vi "loadHTOutcount1.vi"(11 "file (use dialog)":path=path "C:/temp/ht/MachineState/MachineState.txt") -> ()   [LabVIEW 2012]
uses:
  <vilib>/addons/database/Connection.llb/DB Tools Open Connec (Path).vi
  <vilib>/Utility/file.llb/Read From Spreadsheet File (string).vi
  <vilib>/addons/database/Connection.llb/Conn Execute.vi
  <vilib>/addons/database/Recordset.llb/Rec Fetch Integer Data (R).vi
  <vilib>/addons/database/Recordset.llb/Rec Destroy - Connection.vi
  <vilib>/addons/database/NI_Database_API.lvlib
panel:
  out "ToRunSite":string
  out "concatenated string":string
  out "error out 2":errorcluster
  out "SQLDateTime 2":string
  in  "input cluster":T1
  out "output cluster":T1
  out "SQLDateTime":string
  out "time stamp":timestamp
  out "all rows":string[][](array[string])
  out "size(s)":i32[](array[numeric])
  out "error out":errorcluster
  out "output cluster 2":T2
  in  "input cluster 2":T2
  out "before substring 5":string
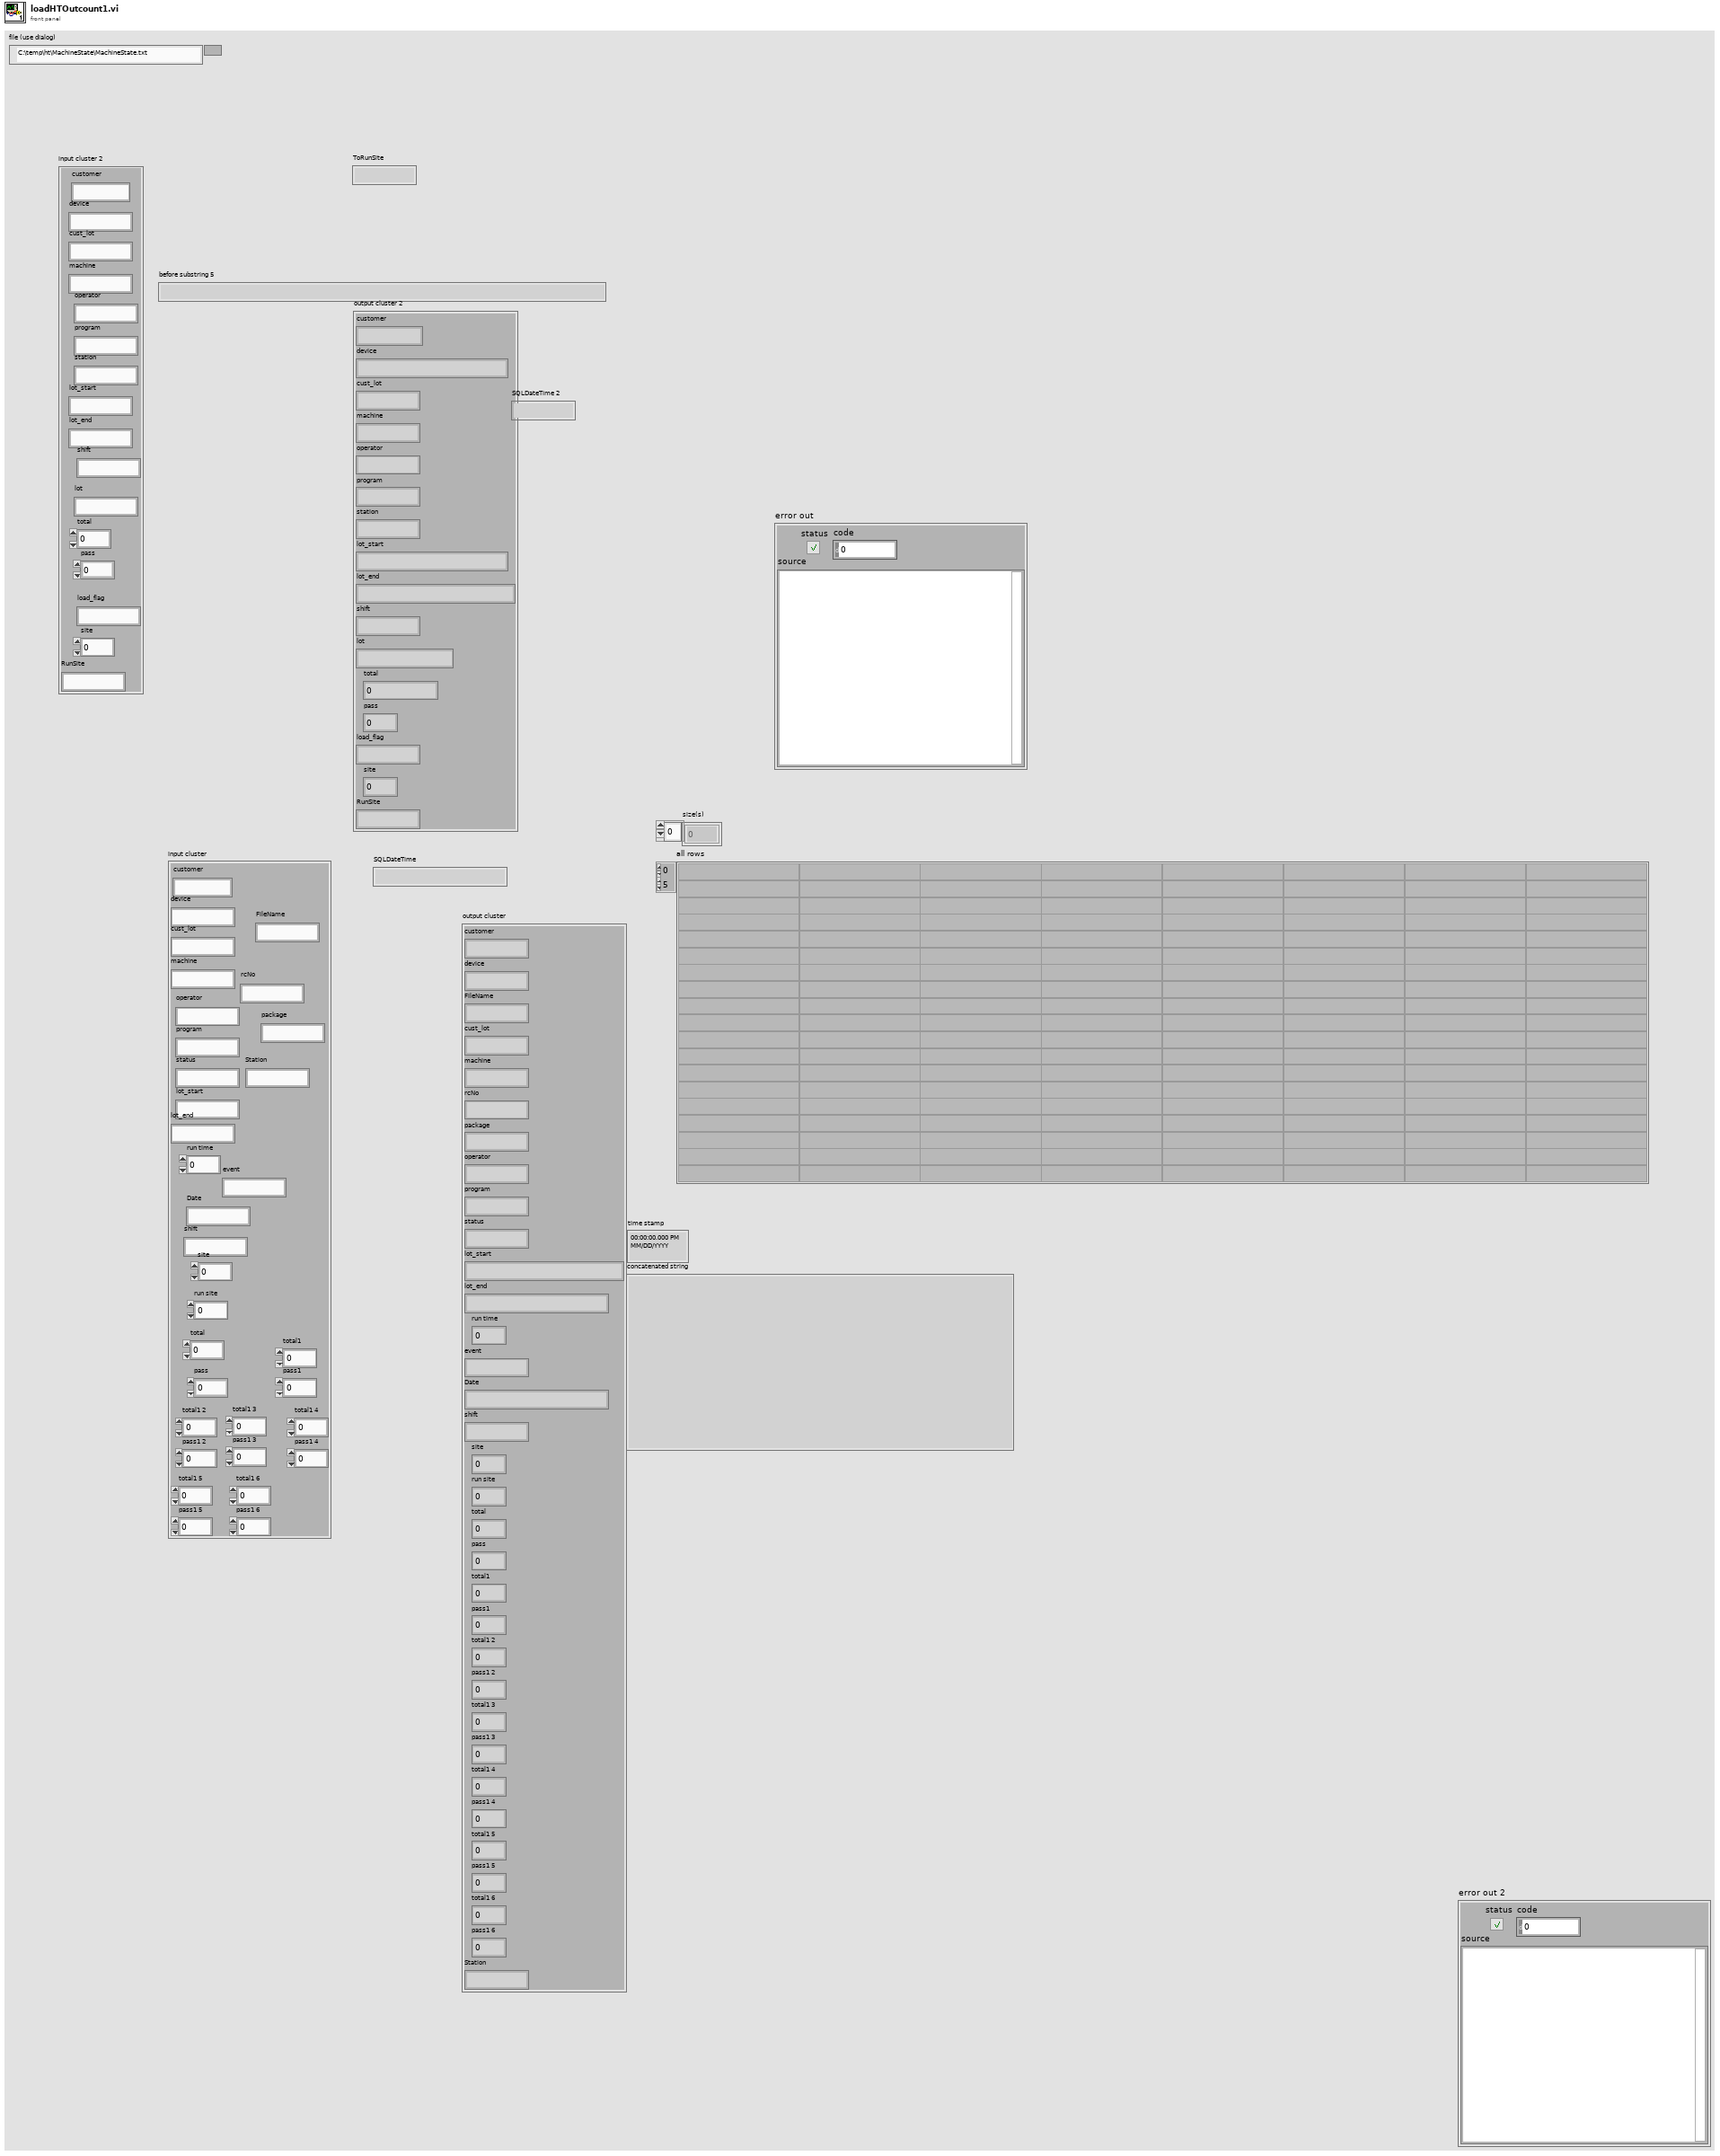
[diagram p1: front panel]
types:
  T1 = cluster{"customer":string, "device":string, "FileName":string, "cust_lot":string, "machine":string, "rcNo":string, "package":string, "operator":string, "program":string, "status":string, "lot_start":string, "lot_end":string, "run time":dbl, "event":string, "Date":string, "shift":string, "site":dbl, "run site ":dbl, "total":dbl, "pass":dbl, "total1":dbl, "pass1":dbl, "total1 2":dbl, "pass1 2":dbl, "total1 3":dbl, "pass1 3":dbl, "total1 4":dbl, "pass1 4":dbl, "total1 5":dbl, "pass1 5":dbl, "total1 6":dbl, "pass1 6":dbl, "Station":string}
  T2 = cluster{"customer":string, "device":string, "cust_lot":string, "machine":string, "operator":string, "program":string, "station":string, "lot_start":string, "lot_end":string, "shift":string, "lot":string, "total":dbl, "pass":dbl, "load_flag":string, "site":dbl, "RunSite":string}
  T3 = typedef "NI_Database_API.lvlib/Conn ObjectReference.ctl" = refnum<k1>
  T4 = typedef "NI_Database_API.lvlib/Rec ObjectReference.ctl" = refnum<k1>
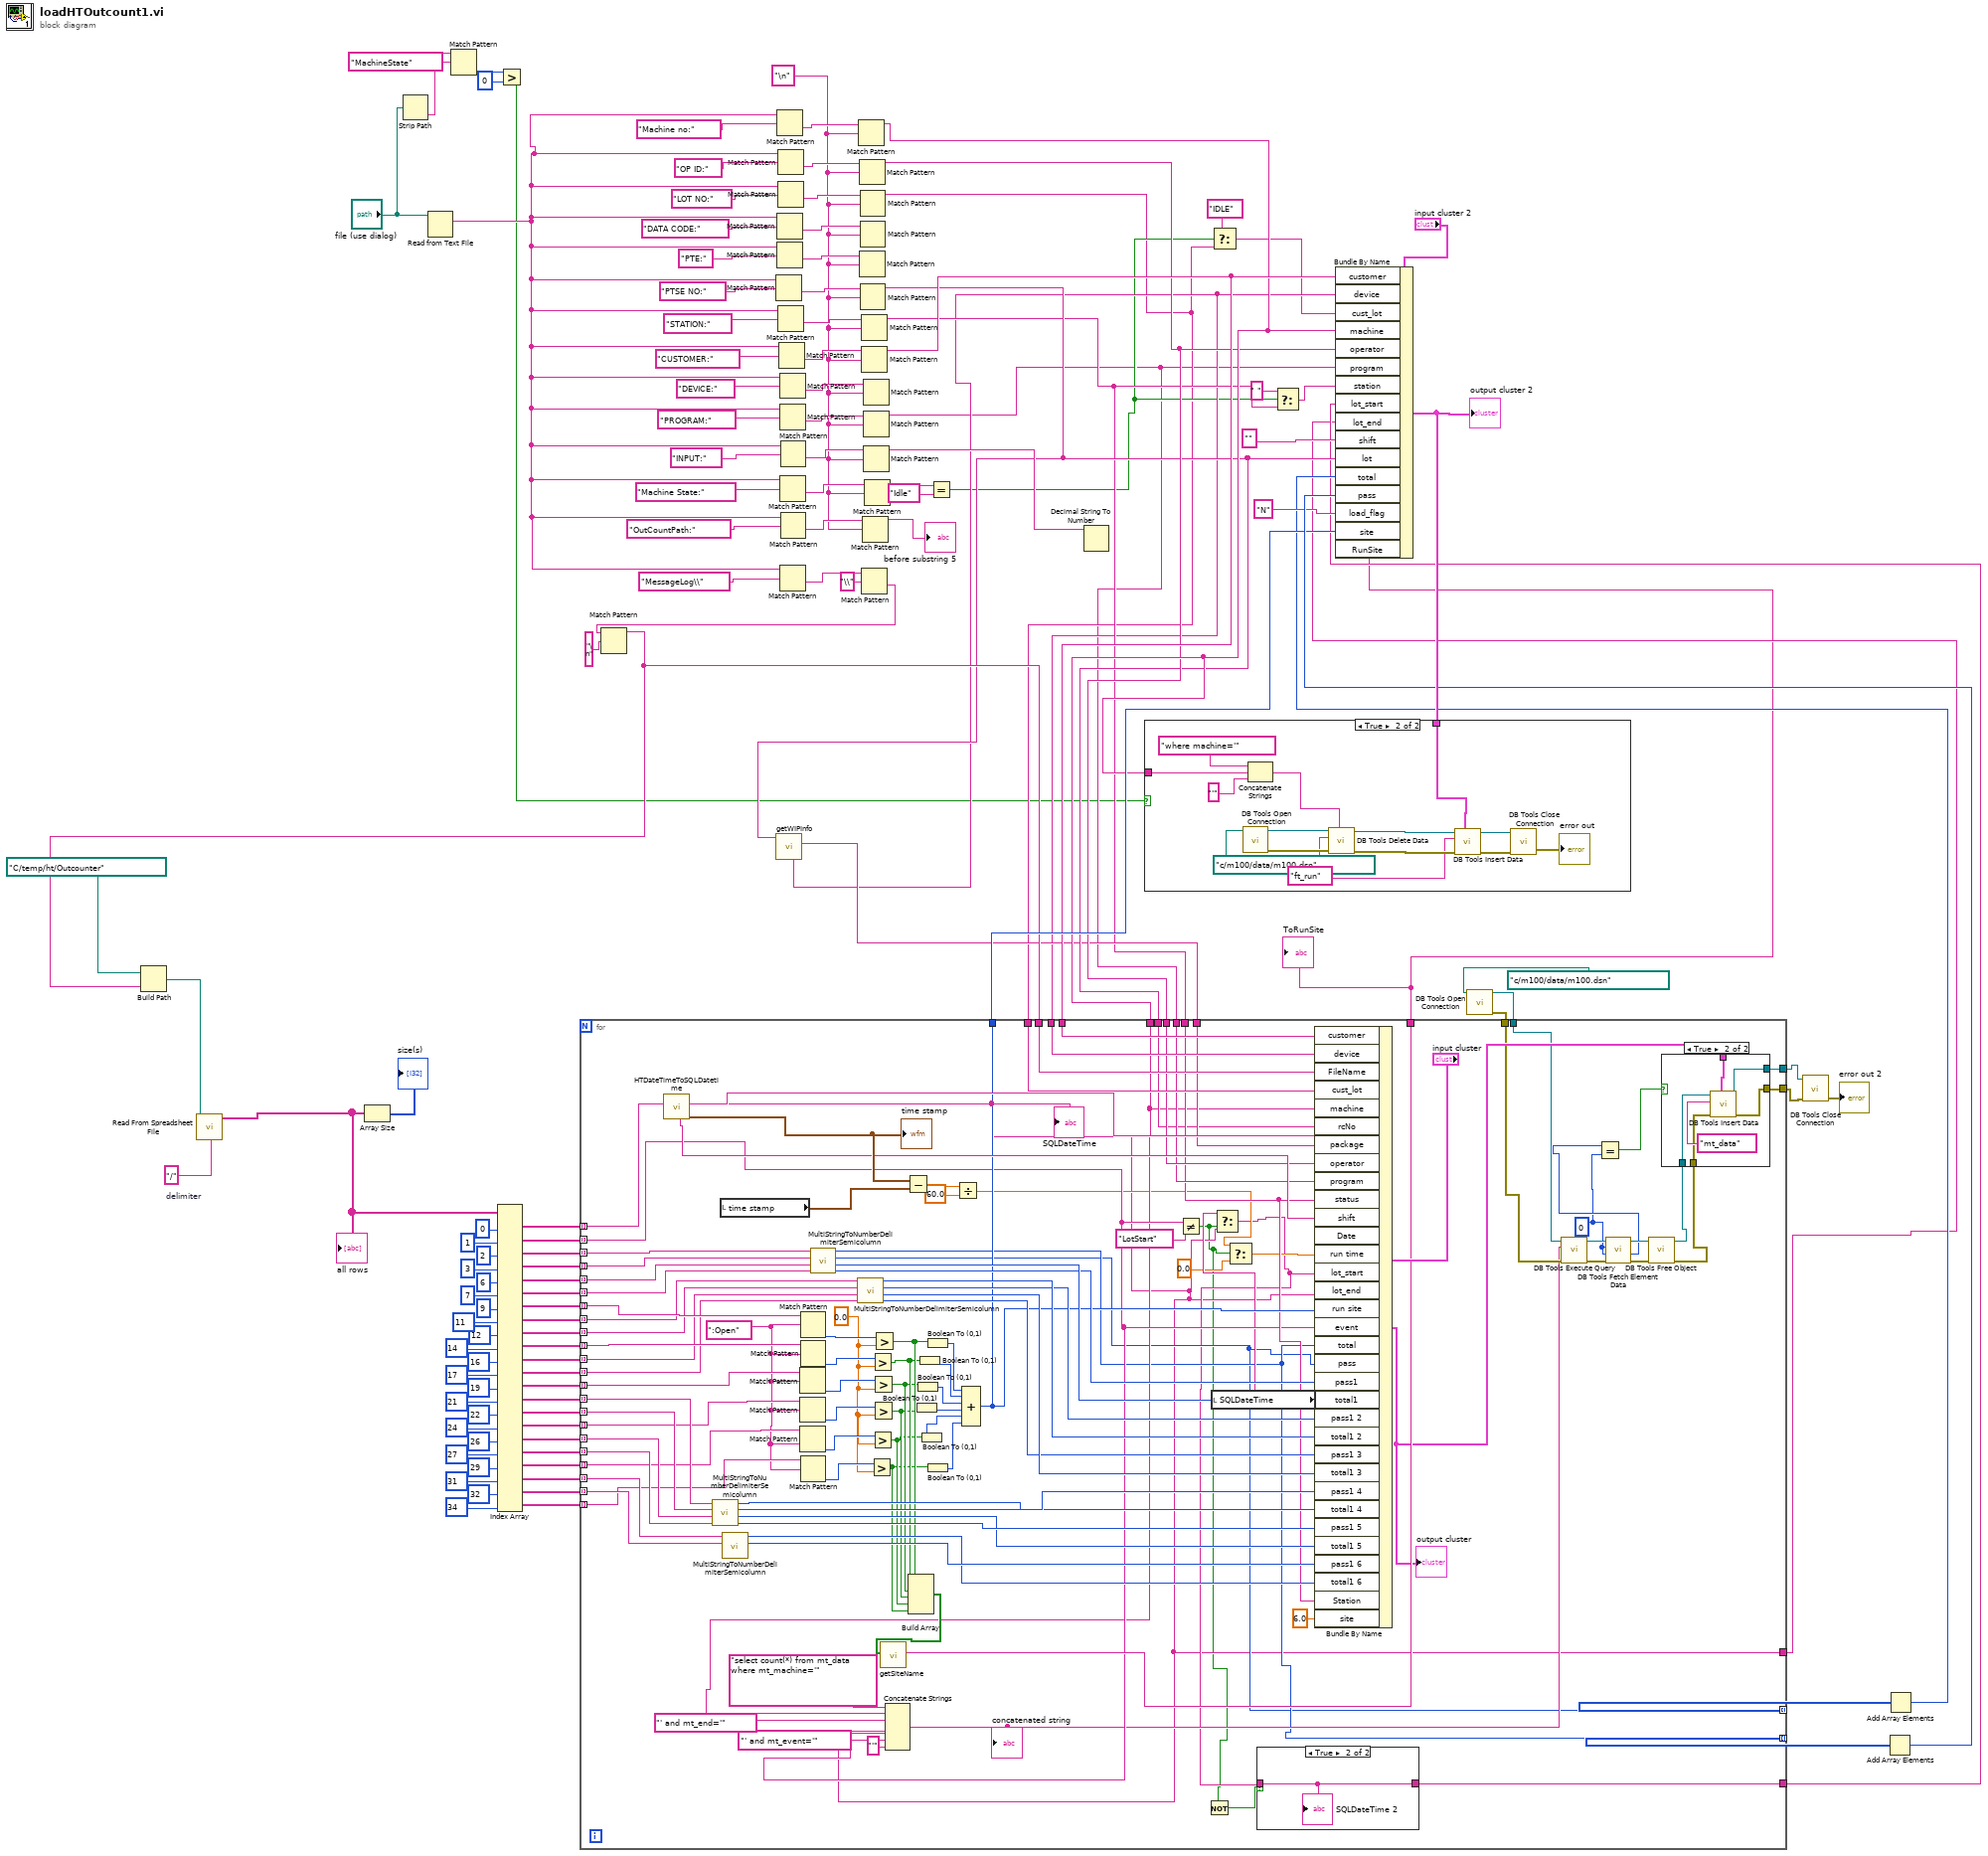
[diagram p0: block diagram]
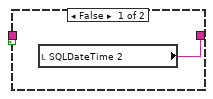
[diagram p4: hidden frame]
diagram:
  w89 = "/"  # delimiter
  w95 = "\n" ("regular expression")
  n1 = Strip Path(path="file (use dialog)") -> (name=w6:string)  [unwired: 1 out]
  n2 = Read from Text File(file (use dialog)="file (use dialog)") -> (text=w92:string)  [unwired: 3 in, 3 out]
  n3 = Match Pattern(string=w6, regular expression="MachineState") -> (offset past match=w4:i32)  [unwired: 1 in, 3 out]
  n4 = Greater?(x=w4, y=0) -> (0:w2:bool)
  n5 = Match Pattern(string=w92, regular expression="PTSE NO:") -> (after substring=w116:string)  [unwired: 1 in, 3 out]
  n6 = Match Pattern(string=w92, regular expression="Machine no:") -> (after substring=w96:string)  [unwired: 1 in, 3 out]
  n7 = Match Pattern(string=w92, regular expression="DATA CODE:") -> (after substring=w120:string)  [unwired: 1 in, 3 out]
  n8 = Match Pattern(string=w92, regular expression="PTE:") -> (after substring=w118:string)  [unwired: 1 in, 3 out]
  n9 = Match Pattern(string=w92, regular expression="OP ID:") -> (after substring=w124:string)  [unwired: 1 in, 3 out]
  n10 = Match Pattern(string=w92, regular expression="LOT NO:") -> (after substring=w122:string)  [unwired: 1 in, 3 out]
  n11 = Match Pattern(string=w92, regular expression="STATION:") -> (after substring=w103:string)  [unwired: 1 in, 3 out]
  n12 = Match Pattern(string=w92, regular expression="CUSTOMER:") -> (after substring=w114:string)  [unwired: 1 in, 3 out]
  n13 = Match Pattern(string=w92, regular expression="DEVICE:") -> (after substring=w112:string)  [unwired: 1 in, 3 out]
  n14 = Match Pattern(string=w92, regular expression="PROGRAM:") -> (after substring=w110:string)  [unwired: 1 in, 3 out]
  n15 = Match Pattern(string=w92, regular expression="Machine State:") -> (after substring=w106:string)  [unwired: 1 in, 3 out]
  n16 = Match Pattern(string=w92, regular expression="MessageLog\\") -> (after substring=w90:string)  [unwired: 1 in, 3 out]
  n17 = Match Pattern(string=w92, regular expression="INPUT:") -> (after substring=w108:string)  [unwired: 1 in, 3 out]
  n18 = Match Pattern(string=w92, regular expression="OutCountPath:") -> (after substring=w104:string)  [unwired: 1 in, 3 out]
  n19 = Match Pattern(string=w96, regular expression=w95) -> (before substring=w30:string)  [unwired: 1 in, 3 out]
  n20 = Match Pattern(string=w124, regular expression=w95) -> (before substring=w29:string)  [unwired: 1 in, 3 out]
  n21 = Match Pattern(string=w118, regular expression=w95) -> ()  [unwired: 1 in, 4 out]
  n22 = Match Pattern(string=w122, regular expression=w95) -> (before substring=w11:string)  [unwired: 1 in, 3 out]
  n23 = Match Pattern(string=w120, regular expression=w95) -> ()  [unwired: 1 in, 4 out]
  n24 = Match Pattern(string=w116, regular expression=w95) -> (before substring=w28:string)  [unwired: 1 in, 3 out]
  n25 = call "getWIPInfo.vi"("Lotno"=w28) -> ("Package"=w27:string, "Product"=w13:string)  [unwired: 4 in, 5 out]
  n26 = Match Pattern(string=w103, regular expression=w95) -> (before substring=w16:string)  [unwired: 1 in, 3 out]
  n27 = Match Pattern(string=w114, regular expression=w95) -> (before substring=w32:string)  [unwired: 1 in, 3 out]
  n28 = Match Pattern(string=w90, regular expression="\\") -> (after substring=w40:string)  [unwired: 1 in, 3 out]
  n29 = Match Pattern(string=w40, regular expression="\n") -> (before substring=w31:string)  [unwired: 1 in, 3 out]
  n30 = Build Path(base path=path "C:/temp/ht/Outcounter", name or relative path=w31) -> (appended path=w41:path)
  n31 = call-poly <vilib>:"Read From Spreadsheet File.vi"("delimiter (\\t)"=w89, "file path (dialog if empty)"=w41) -> ("all rows"=w87:string[][])  [unwired: 5 in, 4 out]
  "all rows" <- w87
  n32 = Array Size(array=w87) -> (size(s)=→"size(s)":i32[])
  n33 = Index Array(array=w87, index (col) #1=0 ("disabled index (col)"), index (col) #2=1 ("index (col)"), index (col) #3=2 ("index (col)"), index (col) #4=3 ("index (col)"), index (col) #5=6 ("index (col)"), index (col) #6=7 ("index (col)"), index (col) #7=9 ("index (col)"), index (col) #8=11 ("index (col)"), index (col) #9=12 ("index (col)"), index (col) #10=14 ("index (col)"), index (col) #11=16 ("index (col)"), index (col) #12=17 ("index (col)"), index (col) #13=19 ("index (col)"), index (col) #14=21 ("index (col)"), index (col) #15=22 ("index (col)"), index (col) #16=24 ("index (col)"), index (col) #17=26 ("index (col)"), index (col) #18=27 ("index (col)"), index (col) #19=29 ("index (col)"), index (col) #20=31 ("index (col)"), index (col) #21=32 ("index (col)"), index (col) #22=34 ("index (col)")) -> (element #1=w85:string[], element #2=w83:string[], element #3=w80:string[], element #4=w79:string[], element #5=w76:string[], element #6=w75:string[], element #7=w73:string[], element #8=w70:string[], element #9=w69:string[], element #10=w67:string[], element #11=w64:string[], element #12=w63:string[], element #13=w61:string[], element #14=w58:string[], element #15=w57:string[], element #16=w55:string[], element #17=w52:string[], element #18=w51:string[], element #19=w49:string[], element #20=w46:string[], element #21=w45:string[], element #22=w43:string[])  [unwired: 22 in]
  n34 = Match Pattern(string=w104, regular expression=w95) -> (before substring=→"before substring 5":string)  [unwired: 1 in, 3 out]
  n35 = Match Pattern(string=w112, regular expression=w95) -> ()  [unwired: 1 in, 4 out]
  n36 = Match Pattern(string=w110, regular expression=w95) -> (before substring=w8:string)  [unwired: 1 in, 3 out]
  n37 = Match Pattern(string=w108, regular expression=w95) -> (before substring=w98:string)  [unwired: 1 in, 3 out]
  n38 = Match Pattern(string=w106, regular expression=w95) -> (before substring=w18:string)  [unwired: 1 in, 3 out]
  n39 = Equal?(x=w18, y="Idle") -> (x = y?=w12:bool)
  n40 = Decimal String To Number(string=w98) -> ()  [unwired: 2 in, 2 out]
  n41 = Select(t="IDLE", s=w12, f=w11) -> (s? t:f=w10:string)
  n42 = Select(t=" ", s=w12, f=w16) -> (s? t:f=w15:string)
  n43 = call-poly <vilib>:"DB Tools Open Connection.vi"("connection information"=path "c:/m100/data/m100.dsn") -> ("error out"=w24:errorcluster, "connection reference"=w25:T3)  [unwired: 7 in]
  n44 = for {
    tunnel: w85 -> [w231] mode=indexing
    tunnel: w83 -> [w151] mode=indexing
    tunnel: w80 -> [w229] mode=indexing
    tunnel: w79 -> [w228] mode=indexing
    tunnel: w76 -> [w227] mode=indexing
    tunnel: w75 -> [w226] mode=indexing
    tunnel: w73 -> [w230] mode=indexing
    tunnel: w70 -> [w225] mode=indexing
    tunnel: w69 -> [w224] mode=indexing
    tunnel: w67 -> [w223] mode=indexing
    tunnel: w64 -> [w222] mode=indexing
    tunnel: w63 -> [w221] mode=indexing
    tunnel: w61 -> [w220] mode=indexing
    tunnel: w58 -> [w219] mode=indexing
    tunnel: w57 -> [w218] mode=indexing
    tunnel: w55 -> [w217] mode=indexing
    tunnel: w52 -> [w216] mode=indexing
    tunnel: w51 -> [w215] mode=indexing
    tunnel: w49 -> [w214] mode=indexing
    tunnel: w46 -> [w213] mode=indexing
    tunnel: w45 -> [w212] mode=indexing
    tunnel: w43 -> [w198] mode=indexing
    tunnel: [w135] -> w38 mode=indexing
    tunnel: [w162] -> w36
    tunnel: [w170] -> w1
    tunnel: [w134] -> w34 mode=indexing
    tunnel: w32 -> [w169]
    tunnel: w13 -> [w168]
    tunnel: w31 -> [w167]
    tunnel: w11 -> [w166]
    tunnel: w30 -> [w138]
    tunnel: w28 -> [w152]
    tunnel: w29 -> [w165]
    tunnel: w8 -> [w164]
    tunnel: w16 -> [w157]
    tunnel: w27 -> [w163]
    tunnel: w25 -> [w146]
    tunnel: w24 -> [w145]
    tunnel: [w161] -> w22
    tunnel: [w160] -> w21
    tunnel: [w130] -> w20
    tunnel: [w129] -> w19
    w142 = 0
    w190 = 0.0 ("y")
    w197 = ":Open" ("regular expression")
    n45 = call "HTDateTimeToSQLDatetime.vi"("HTDateTime"=w231) -> ("time stamp"=w182:timestamp, "date string"=w179:string, "SQLDateTime"=w129:string, "Shift"=w178:string)  [unwired: 7 in]
    "SQLDateTime" <- w129
    "time stamp" <- w182
    n46 = call "MultiStringToNumberDelimiterSemicolumn.vi"("input string 4"=w215, "input string 3"=w216, "input string 2"=w218, "input string"=w219) -> ("number 4"=w208:i32, "number 3"=w207:i32, "number 2"=w206:i32, "number"=w205:i32)  [unwired: 4 in]
    n47 = local read "time stamp"() -> (w183:timestamp)
    n48 = call "MultiStringToNumberDelimiterSemicolumn.vi"("input string 2"=w212, "input string"=w213) -> ("number 2"=w210:i32, "number"=w209:i32)  [unwired: 6 in, 2 out]
    n49 = Match Pattern(string=w220, regular expression=w197) -> (offset past match=w194:i32)  [unwired: 1 in, 3 out]
    n50 = Match Pattern(string=w217, regular expression=w197) -> (offset past match=w193:i32)  [unwired: 1 in, 3 out]
    n51 = Match Pattern(string=w214, regular expression=w197) -> (offset past match=w192:i32)  [unwired: 1 in, 3 out]
    n52 = Match Pattern(string=w230, regular expression=w197) -> (offset past match=w196:i32)  [unwired: 1 in, 3 out]
    n53 = Match Pattern(string=w223, regular expression=w197) -> (offset past match=w195:i32)  [unwired: 1 in, 3 out]
    n54 = Match Pattern(string=w198, regular expression=w197) -> (offset past match=w191:i32)  [unwired: 1 in, 3 out]
    n55 = call "MultiStringToNumberDelimiterSemicolumn.vi"("input string 4"=w226, "input string 3"=w227, "input string 2"=w228, "input string"=w229) -> ("number 4"=w199:i32, "number 3"=w200:i32, "number 2"=w134:i32, "number"=w135:i32)  [unwired: 4 in]
    n56 = call "MultiStringToNumberDelimiterSemicolumn.vi"("input string 4"=w221, "input string 3"=w222, "input string 2"=w224, "input string"=w225) -> ("number 4"=w203:i32, "number 3"=w204:i32, "number 2"=w201:i32, "number"=w202:i32)  [unwired: 4 in]
    n57 = Greater?(x=w191, y=w190) -> (0:w172:bool)
    n58 = Greater?(x=w195, y=w190) -> (0:w176:bool)
    n59 = Greater?(x=w192, y=w190) -> (0:w173:bool)
    n60 = Greater?(x=w194, y=w190) -> (0:w175:bool)
    n61 = Greater?(x=w193, y=w190) -> (0:w174:bool)
    n62 = Greater?(x=w196, y=w190) -> (0:w177:bool)
    n63 = Concatenate Strings("select count(*) from mt_data where mt_machine='" ("string"), w138, "' and mt_end='" ("string"), w129, "' and mt_event='" ("string"), w151, "'" ("string")) -> (w144:string)
    "concatenated string" <- w144
    n64 = Subtract(x=w182, y=w183) -> (x-y=w181:dbl)
    n65 = Build Array(w177, w176, w175, w174, w173, w172) -> (w171:bool[])
    n66 = call "getSiteName.vi"("Array"=w171) -> ("String"=w170:string)  [unwired: 10 in]
    n67 = Boolean To (0,1)(Boolean=w174) -> (0, 1=w186:i16)
    n68 = Boolean To (0,1)(Boolean=w175) -> (0, 1=w187:i16)
    n69 = Boolean To (0,1)(Boolean=w176) -> (0, 1=w188:i16)
    n70 = Boolean To (0,1)(Boolean=w173) -> (0, 1=w185:i16)
    n71 = Boolean To (0,1)(Boolean=w177) -> (0, 1=w189:i16)
    n72 = Boolean To (0,1)(Boolean=w172) -> (0, 1=w184:i16)
    n73 = Divide(x=w181, y=60.0) -> (x/y=w133:dbl)
    n74 = Compound Arithmetic op=ADD(w189, w188, w187, w186, w185, w184) -> (w162:i16)
    n75 = Not Equal?(x=w151, y="LotStart") -> (x != y?=w127:bool)
    n76 = Not(x=w127) -> (.not. x?=w126:bool)
    n77 = local read "SQLDateTime"() -> (w136:string)
    n78 = Select(t=w136, s=w127, f=w129) -> (s? t:f=w131:string)
    n79 = Select(t=w133, s=w127, f=0.0 ("t")) -> (s? t:f=w137:dbl)
    n80 = case shown="True" w126 {
      tunnel: w131 -> [_ w241]
      tunnel: [w240 w241] -> w130
      frame False {
        n81 = local read "SQLDateTime 2"() -> (w240:string)
      }
      frame True {
        "SQLDateTime 2" <- w241
      }
    }
    n82 = Bundle By Name(cluster="input cluster", "customer"=w169, "device"=w168, "FileName"=w167, "cust_lot"=w166, "machine"=w138, "rcNo"=w152, "package"=w163, "operator"=w165, "program"=w164, "status"=w157, "shift"=w178, "Date"=w179, "run time"=w137, "lot_start"=w131, "lot_end"=w129, "run site"=w162, "event"=w151, "total"=w135, "pass"=w134, "pass1"=w199, "total1"=w200, "pass1 2"=w201, "total1 2"=w202, "pass1 3"=w203, "total1 3"=w204, "pass1 4"=w206, "total1 4"=w205, "pass1 5"=w208, "total1 5"=w207, "pass1 6"=w210, "total1 6"=w209, "Station"=w157, "site"=6.0) -> (w159:T1)
    "output cluster" <- w159
    n83 = call-poly <vilib>:"DB Tools Execute Query.vi"("error in (no error)"=w145, "SQL query"=w144, "connection reference"=w146) -> ("error out"=w150:errorcluster, "recordset reference"=w149:T4)  [unwired: 5 in]
    n84 = call-poly <vilib>:"DB Tools Fetch Element Data.vi"("error in (no error)"=w150, "type"=w142, "column index"=w142, "recordset reference"=w149) -> ("error out"=w148:errorcluster, "data"=w143:i32, "recordset reference out"=w147:T4)  [unwired: 3 in]
    n85 = Equal?(x=w143, y=w142) -> (x = y?=w141:bool)
    n86 = call-poly <vilib>:"DB Tools Free Object.vi"("error in (no error)"=w148, "recordset reference"=w147) -> ("error out"=w139:errorcluster, "connection reference"=w140:T3)  [unwired: 8 in]
    n87 = case shown="True" w141 {
      tunnel: [w233 w239] -> w161
      tunnel: [w232 w238] -> w160
      tunnel: w159 -> [_ w236]
      tunnel: w140 -> [w233 w235]
      tunnel: w139 -> [w232 w234]
      frame False {
      }
      frame True {
        n88 = call <vilib>:"DB Tools Insert Data.vi"("data"=w236, "error in (no error)"=w234, "table"="mt_data", "connection reference"=w235) -> ("error out"=w238:errorcluster, "connection reference out"=w239:T3)  [unwired: 6 in]
      }
    }
  }
  "ToRunSite" <- w1
  n89 = call <vilib>:"DB Tools Close Connection.vi"("error in (no error)"=w21, "connection reference"=w22) -> ("error out"=→"error out 2":errorcluster)  [unwired: 5 in]
  n90 = Add Array Elements(numeric array=w38) -> (sum=w37:i32)
  n91 = Add Array Elements(numeric array=w34) -> (sum=w33:i32)
  n92 = Bundle By Name(cluster="input cluster 2", "customer"=w32, "device"=w13, "cust_lot"=w10, "machine"=w30, "operator"=w29, "program"=w8, "station"=w15, "lot_start"=w20, "lot_end"=w19, "shift"="" ("lot_end"), "lot"=w28, "total"=w33, "pass"=w37, "load_flag"="N", "site"=w36, "RunSite"=w1) -> (w94:T2)
  "output cluster 2" <- w94
  n93 = case shown="True" w2 {
    tunnel: w94 -> [_ w246]
    tunnel: w30 -> [_ w244]
    frame False {
    }
    frame True {
      w245 = "ft_run" ("table")
      n94 = call-poly <vilib>:"DB Tools Open Connection.vi"("connection information"=path "c:/m100/data/m100.dsn") -> ("error out"=w254:errorcluster, "connection reference"=w255:T3)  [unwired: 7 in]
      n95 = Concatenate Strings("where machine='" ("string"), w244, "'" ("string")) -> (w250:string)
      n96 = call <vilib>:"DB Tools Delete Data.vi"("condition"=w250, "error in (no error)"=w254, "table"=w245, "connection reference"=w255) -> ("error out"=w247:errorcluster, "connection reference out"=w248:T3)  [unwired: 6 in]
      n97 = call <vilib>:"DB Tools Insert Data.vi"("data"=w246, "error in (no error)"=w247, "table"=w245, "connection reference"=w248) -> ("error out"=w242:errorcluster, "connection reference out"=w243:T3)  [unwired: 6 in]
      n98 = call <vilib>:"DB Tools Close Connection.vi"("error in (no error)"=w242, "connection reference"=w243) -> ("error out"=→"error out":errorcluster)  [unwired: 5 in]
    }
  }
